vi "TYPE.vi"(8 "error in (no error)":errorcluster, 10 "Type":u16(ring) items=["ASCII", "Binary"], 11 "FTP in":refnum<class "FTP.lvclass">) -> (0 "error out":errorcluster, 3 "FTP out":refnum<class "FTP.lvclass">)   [LabVIEW 2017, in "FTP.lvlib" / "FTP.lvclass"]
uses:
  FTP.lvclass
panel:
  out "Line":string
  out "code":i32
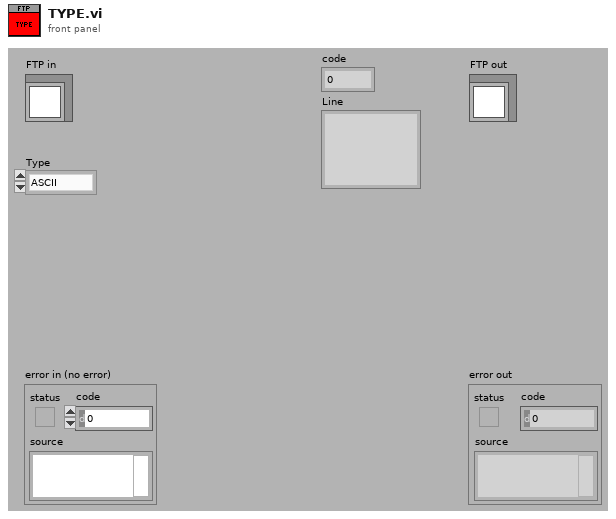
[diagram p1: front panel]
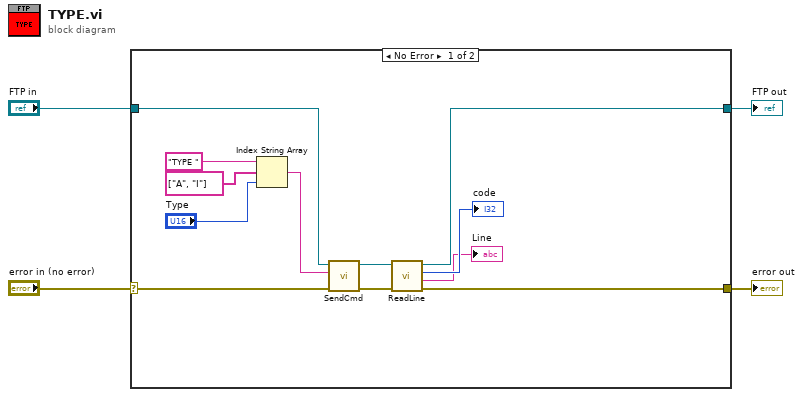
[diagram p0: block diagram]
diagram:
  n1 = case shown="No Error" "error in (no error)" {
    selector: "error in (no error)" -> [w12 w18]
    tunnel: [w11 w18] -> w3
    tunnel: [w13 w17] -> w1
    tunnel: "FTP in" -> [w14 w17]
    frame No Error {
      n2 = Index String Array(1:"Type", 2:string[] ["A", "I"], 3:"TYPE " ("cmd")) -> (0:w10:string)
      n3 = call "SendCmd.vi"("error in (no error)"=w12, "cmd"=w10, "FTP in"=w14) -> ("error out"=w15:errorcluster, "FTP out"=w16:refnum<class "FTP.lvclass">)  [unwired: 7 in]
      n4 = call "ReadLine.vi"("error in (no error)"=w15, "FTP in"=w16) -> ("error out"=w11:errorcluster, "Line"=→"Line":string, "code"=→"code":i32, "FTP out"=w13:refnum<class "FTP.lvclass">)  [unwired: 5 in, 1 out]
    }
    frame Error {
    }
  }
  "error out" <- w3
  "FTP out" <- w1
